vi "StopVI.vi"(0 "Application Ref in":refnum<vi>, 5 "VI in":refnum<vi>, 11 "error in (no error)":errorcluster) -> (15 "error out":errorcluster)   [LabVIEW 2016]
uses:
  main/apis/Stimulus/ValueSignal/ValueSignalByPathString.vi
  main/Drona.lvlib
  main/apis/Stimulus/ValueSignal/ValueSignal.lvlib
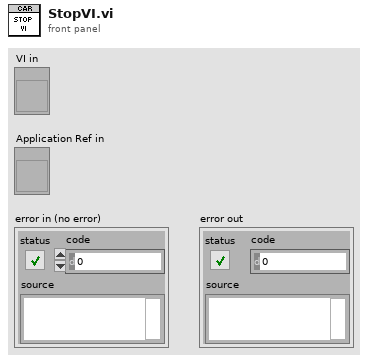
[diagram p1: front panel]
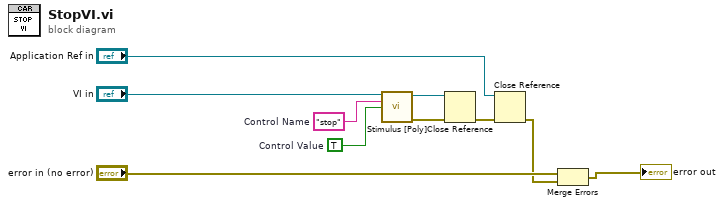
[diagram p0: block diagram]
diagram:
  w5 = TRUE  # Control Value
  w6 = "stop"  # Control Name
  n1 = call-poly "Stimulus [Poly].vi"("VI Reference In"="VI in", "Control Path"=w6, "Value (Signaling)"=w5) -> ("VI Reference Out"=w2:refnum<vi>, "error out"=w4:errorcluster)  [unwired: 11 in]
  n2 = Close Reference(reference=w2, error in (no error)=w4) -> (error out=w3:errorcluster)
  n3 = Close Reference(reference="Application Ref in", error in (no error)=w3) -> (error out=w1:errorcluster)
  n4 = Merge Errors("error in (no error)", w1) -> (→"error out":errorcluster)
